vi "Camera Rotation.vi"(11 "Auto Stack":bool) -> ()   [LabVIEW 2014]
uses:
  TypeDefs/SRE Enum.ctl
  Support Code/Robot Global Data.vi
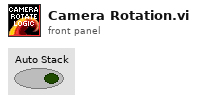
[diagram p1: front panel]
types:
  T1 = typedef "SRE Enum.ctl" = enum16{"Start", "Run", "End"}
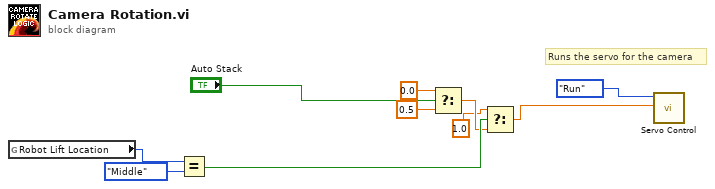
[diagram p0: block diagram]
diagram:
  # "Runs the servo for the camera"
  n1 = global read "Robot Global Data.vi" "Robot Lift Location"() -> (w10:enum16{"High", "Middle", "Low", "Really Low"})
  n2 = Equal?(x=w10, y=enum16{"High", "Middle", "Low", "Really Low"}."Middle") -> (x = y?=w6:bool)
  n3 = Select(t=0.0, s="Auto Stack", f=0.5) -> (s? t:f=w3:dbl)
  n4 = Select(t=1.0 ("f"), s=w6, f=w3) -> (s? t:f=w5:dbl)
  n5 = call "Servo Control.vi"("Position"=w5, "Enum"=SRE_Enum."Run") -> ()  [unwired: 10 in]
